vi "Get Grating.vi"(8 "error in (no error)":errorcluster, 11 "Abstract Spectrometer in":refnum<class "Abstract Spectrometer.lvclass">) -> (0 "error out":errorcluster, 2 "Grating ID":u32, 3 "Abstract Spectrometer out":refnum<class "Abstract Spectrometer.lvclass">)   [LabVIEW 2019, in "Abstract Spectrometer.lvclass"]
uses:
  Abstract Spectrometer.lvclass
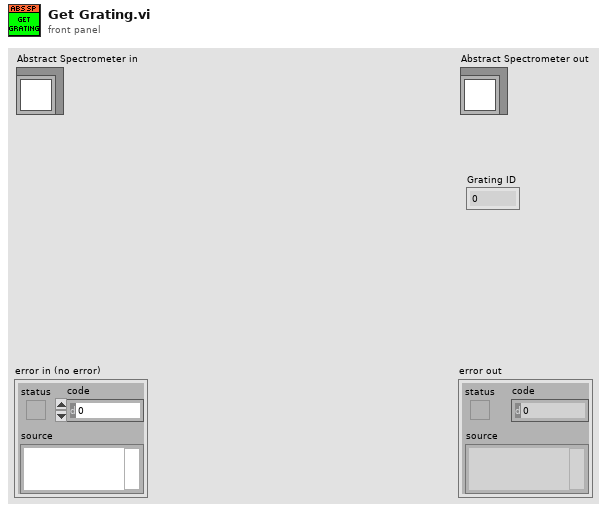
[diagram p1: front panel]
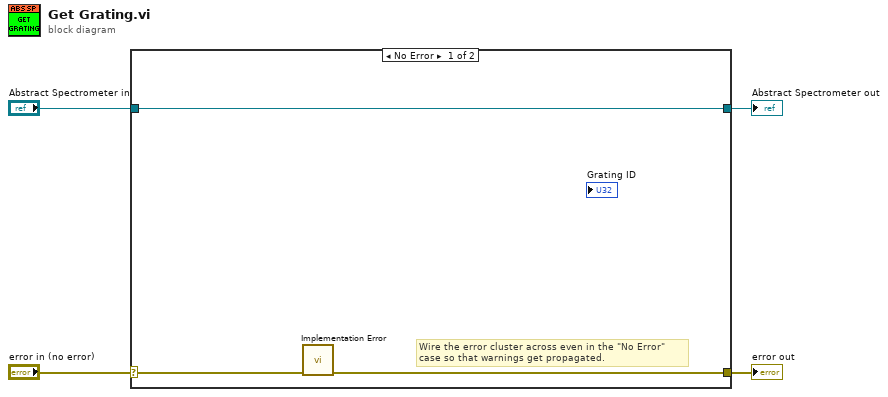
[diagram p0: block diagram]
diagram:
  n1 = case shown="No Error" "error in (no error)" {
    selector: "error in (no error)" -> [w6 w9]
    tunnel: [w5 w9] -> w3
    tunnel: [w7 w8] -> w1
    tunnel: "Abstract Spectrometer in" -> [w7 w8]
    frame No Error {
      # "Wire the error cluster across even in the \"No Error\"\ncase so that warnings get propagated."
      n2 = call "Implementation Error.vi"("error in (no error)"=w6) -> ("error out"=w5:errorcluster)  [unwired: 10 in]
    }
    frame Error {
    }
  }
  "error out" <- w3
  "Abstract Spectrometer out" <- w1
